vi "数据库1操作.vi"(1 "模糊查找内容":string) -> ()   [LabVIEW 2018]
uses:
  <vilib>/Utility/file.llb/Write To Spreadsheet File (string).vi
panel:
  out "error out 3":errorcluster
  out "error out 2":errorcluster
  in  "选项卡控件":enum32{"读取", "写入", "其他"}(tab)
  in  "保存":bool
  in  "查找":bool
  out "Table":string[][](table) caption="表格"
  in  "查找项目":u16(ring) items=["编号", "名称", "零件号", "图号", "批号"]
  in  "数据库所在位置":path
  in  "userID":string="admin"
  in  "userPWD":string="admin"
  in  "以编号写其他":bool
  in  "时间":string="000007"
  in  "批号":string="000006"
  in  "数量":string="000005"
  in  "图号":string="000004"
  in  "零件号":string="000003"
  in  "名称":string="000002"
  in  "插入编号":string="000001"
  in  "插入编号":bool
  out "error out":errorcluster
  # "vi所在文件夹"
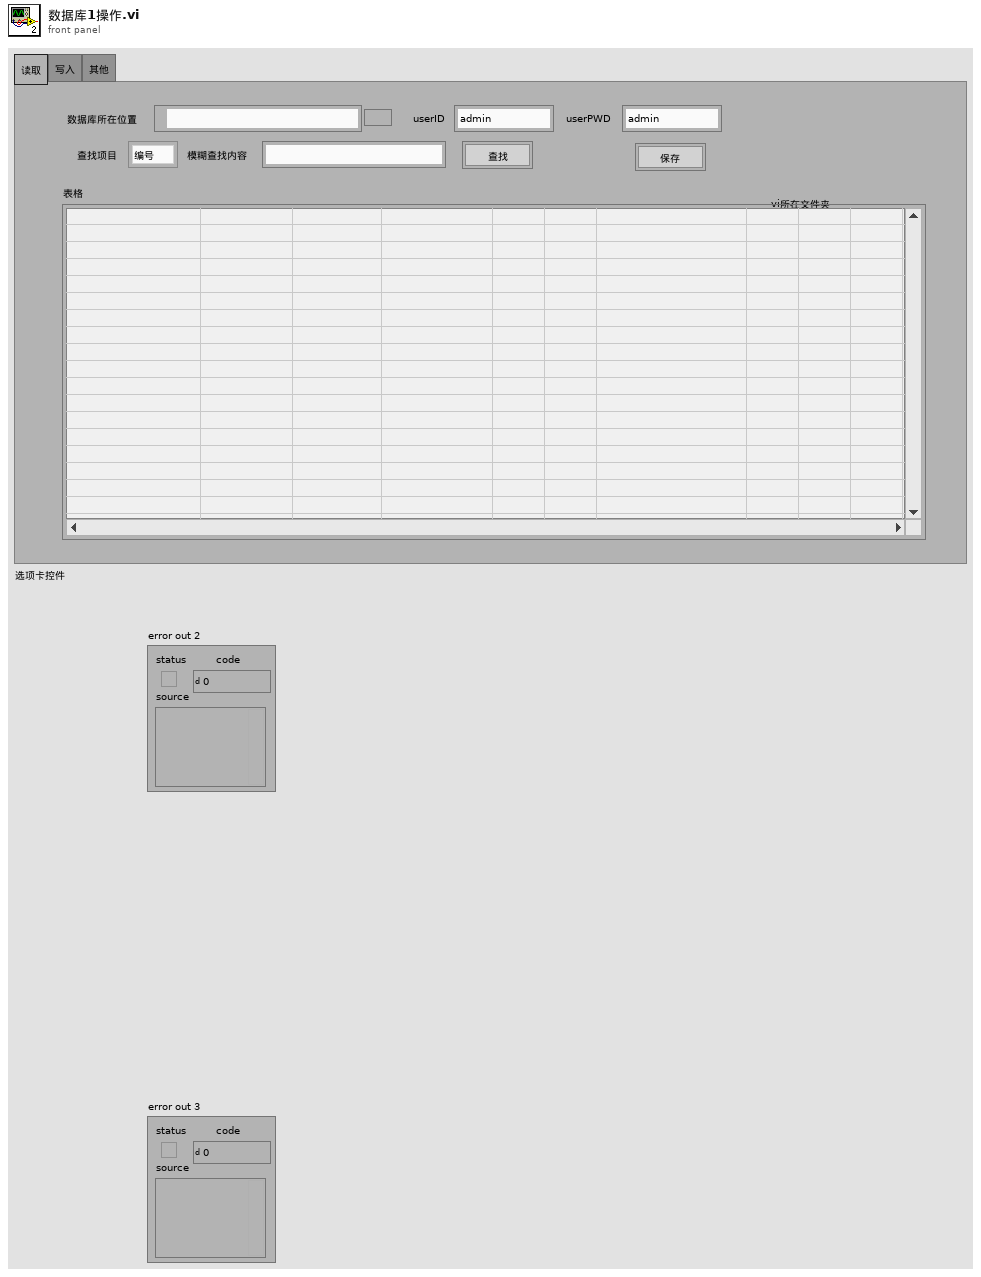
[diagram p1: front panel]
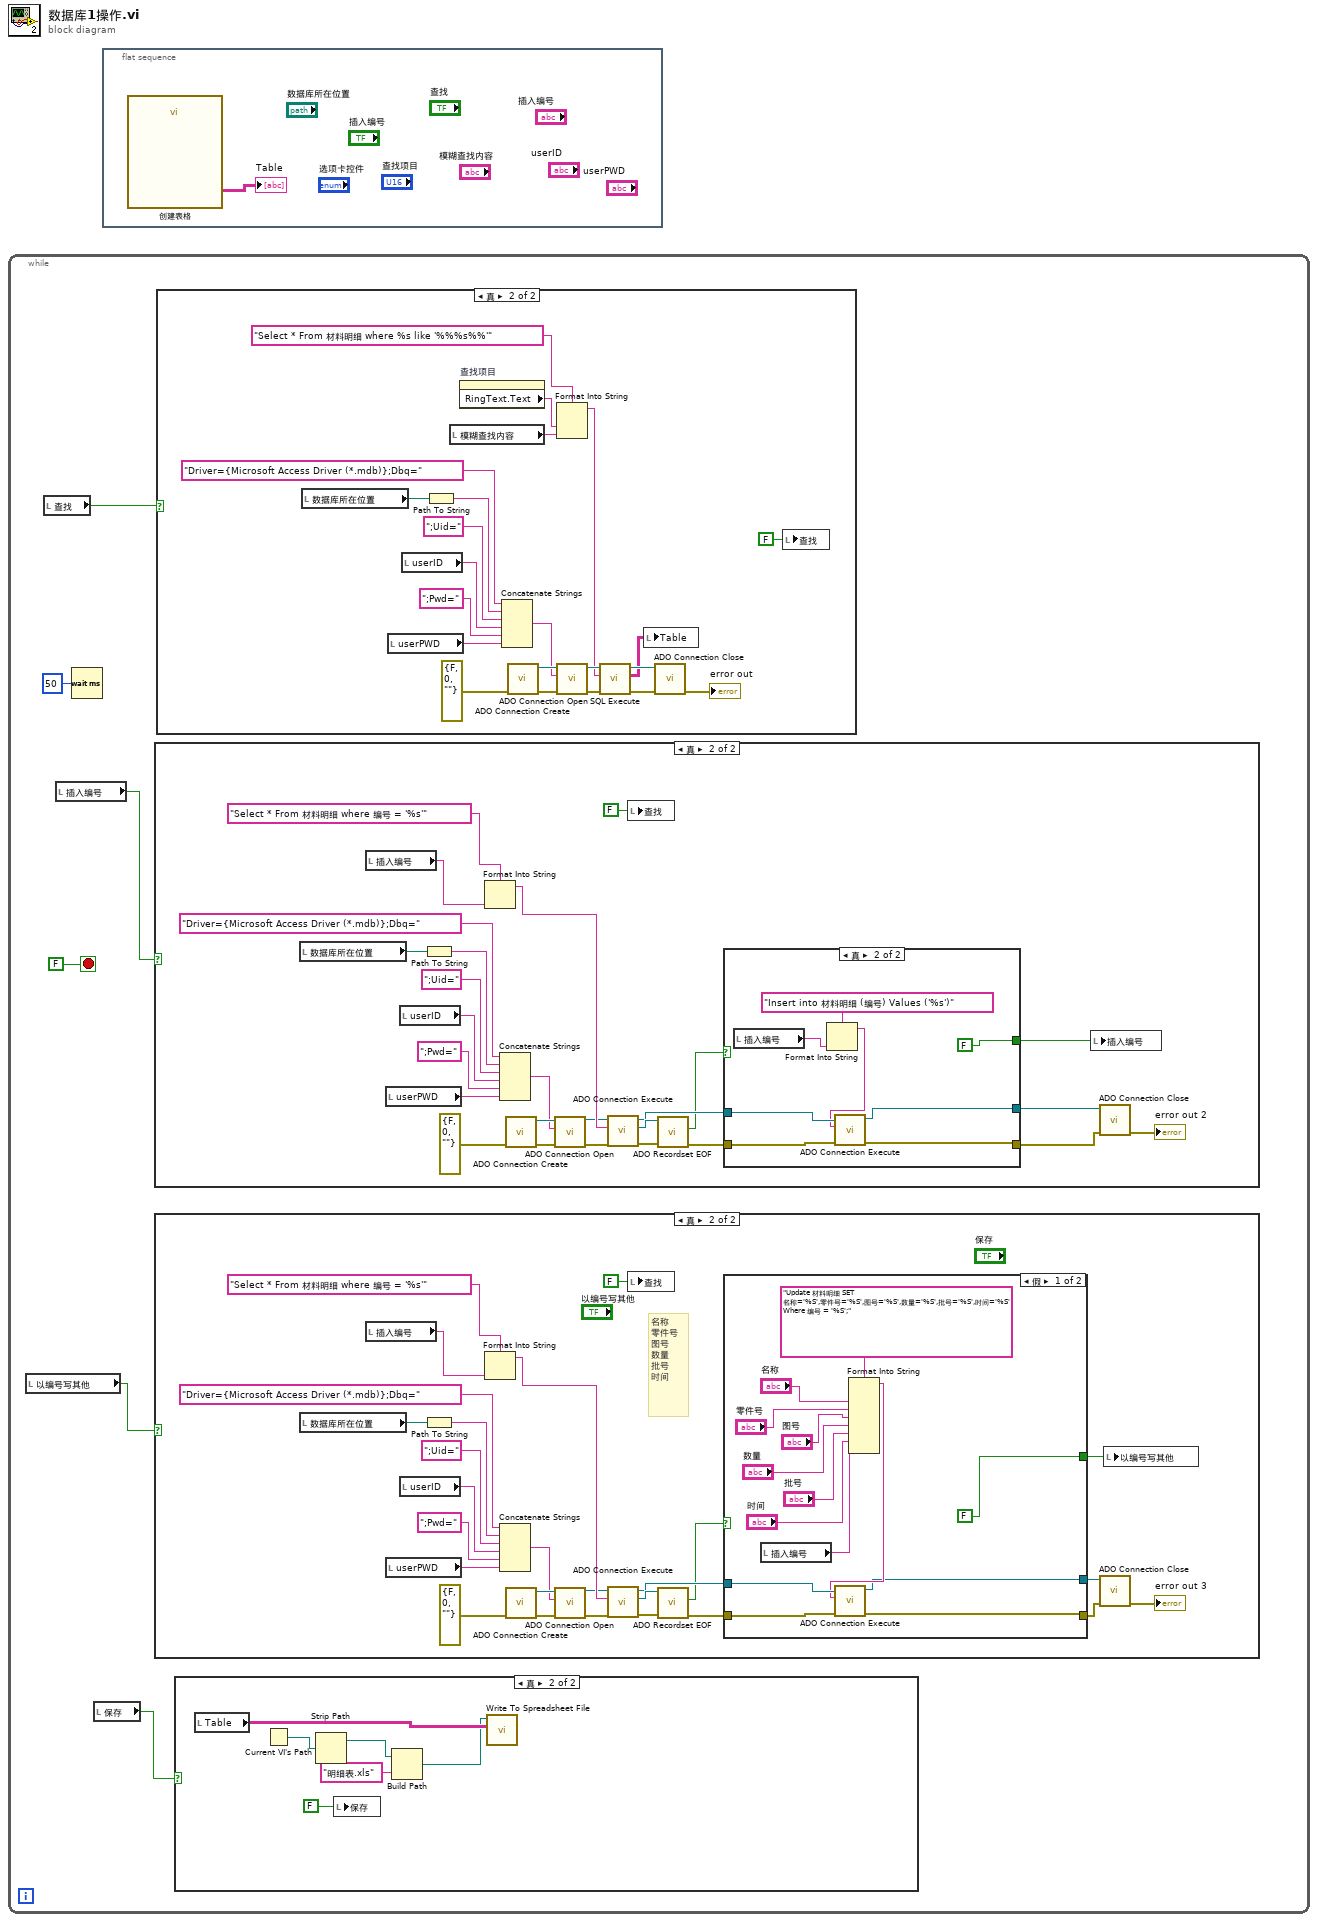
[diagram p0: block diagram]
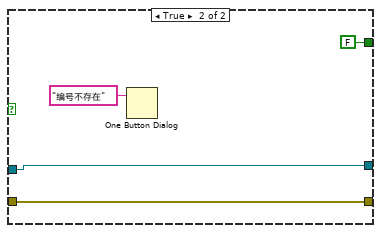
[diagram p4: hidden frame]
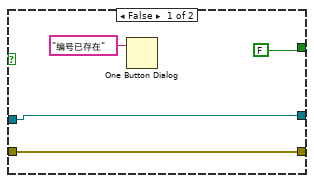
[diagram p6: hidden frame]
diagram:
  n1 = while {
    stop <- FALSE stop-if-true
    n2 = local read "以编号写其他"() -> (w2:bool)
    n3 = local read "查找"() -> (w6:bool)
    n4 = local read "插入编号"() -> (w3:bool)
    n5 = Wait (ms)(milliseconds to wait=u32 50 ("等待时间（毫秒）")) -> ()  [unwired: 1 out]
    n6 = local read "保存"() -> (w1:bool)
    n7 = case shown="真" w3 {
      frame False {
      }
      frame True {
        n8 = local read "数据库所在位置"() -> (w72:path)
        n9 = local read "插入编号"() -> (w68:string)
        n10 = local read "userPWD"() -> (w71:string)
        n11 = local read "userID"() -> (w73:string)
        n12 = Path To String(path=w72) -> (string=w76:string)
        n13 = Format Into String(format string="Select * From 材料明细 where 编号 = '%s'" ("格式字符串"), w68) -> (resulting string=w67:string)  [unwired: 2 in, 1 out]
        n14 = Concatenate Strings("Driver={Microsoft Access Driver (*.mdb)};Dbq=", w76, ";Uid=", w73, ";Pwd=", w71) -> (w77:string)
        n15 = call "ADO Connection Create.vi"("error in (no error)"=errorcluster {"status"=FALSE, "code"=0, "source"=""}) -> ("error out"=w81:errorcluster, "ADODB._Connection Out"=w82:refnum<k7>)  [unwired: 9 out]
        n16 = call "ADO Connection Open.vi"("error in (no error)"=w81, "ConnectionString"=w77, "ADODB._Connection In"=w82) -> ("error out"=w64:errorcluster, "ADODB._Connection Out"=w66:refnum<k7>)  [unwired: 7 out]
        n17 = call "ADO Connection Execute.vi"("error in (no error)"=w64, "CommandText"=w67, "ADODB._Connection In"=w66) -> ("error out"=w63:errorcluster, "RecordSet"=w65:refnum<k7>, "ADODB._Connection Out"=w61:refnum<k7>)  [unwired: 6 in]
        n18 = local write "查找"(FALSE ("读取")) -> ()
        n19 = call "ADO Recordset EOF.vi"("error in (no error)"=w63, "ADODB._Recordset In"=w65) -> ("error out"=w62:errorcluster, "EOF"=w60:bool)  [unwired: 7 in, 1 out]
        n20 = case shown="真" w60 {
          tunnel: w62 -> [w85 w93]
          tunnel: w61 -> [w86 w92]
          tunnel: [w86 w90] -> w59
          tunnel: [w85 w89] -> w58
          tunnel: [FALSE FALSE] -> w57
          frame False {
            n21 = One Button Dialog(message="编号已存在" ("消息")) -> ()  [unwired: 1 in, 1 out]
          }
          frame True {
            n22 = local read "插入编号"() -> (w88:string)
            n23 = Format Into String(format string="Insert into 材料明细 (编号) Values ('%s')" ("格式字符串"), w88) -> (resulting string=w91:string)  [unwired: 2 in, 1 out]
            n24 = call "ADO Connection Execute.vi"("error in (no error)"=w93, "CommandText"=w91, "ADODB._Connection In"=w92) -> ("error out"=w89:errorcluster, "ADODB._Connection Out"=w90:refnum<k7>)  [unwired: 6 in, 1 out]
          }
        }
        n25 = local write "插入编号"(w57) -> ()
        n26 = call "ADO Connection Close.vi"("error in (no error)"=w58, "ADODB._Connection In"=w59) -> ("error out"=→"error out 2":errorcluster)  [unwired: 9 out]
      }
    }
    n27 = case shown="真" w2 {
      frame False {
      }
      frame True {
        # "名称\n零件号\n图号\n数量\n批号\n时间"
        n28 = local read "数据库所在位置"() -> (w28:path)
        n29 = local read "插入编号"() -> (w24:string)
        n30 = local read "userPWD"() -> (w27:string)
        n31 = local read "userID"() -> (w29:string)
        n32 = Path To String(path=w28) -> (string=w32:string)
        n33 = Format Into String(format string="Select * From 材料明细 where 编号 = '%s'" ("格式字符串"), w24) -> (resulting string=w23:string)  [unwired: 2 in, 1 out]
        n34 = Concatenate Strings("Driver={Microsoft Access Driver (*.mdb)};Dbq=", w32, ";Uid=", w29, ";Pwd=", w27) -> (w33:string)
        n35 = call "ADO Connection Create.vi"("error in (no error)"=errorcluster {"status"=FALSE, "code"=0, "source"=""}) -> ("error out"=w37:errorcluster, "ADODB._Connection Out"=w38:refnum<k7>)  [unwired: 9 out]
        n36 = call "ADO Connection Open.vi"("error in (no error)"=w37, "ConnectionString"=w33, "ADODB._Connection In"=w38) -> ("error out"=w20:errorcluster, "ADODB._Connection Out"=w22:refnum<k7>)  [unwired: 7 out]
        n37 = call "ADO Connection Execute.vi"("error in (no error)"=w20, "CommandText"=w23, "ADODB._Connection In"=w22) -> ("error out"=w19:errorcluster, "RecordSet"=w21:refnum<k7>, "ADODB._Connection Out"=w17:refnum<k7>)  [unwired: 6 in]
        n38 = local write "查找"(FALSE ("读取")) -> ()
        n39 = call "ADO Recordset EOF.vi"("error in (no error)"=w19, "ADODB._Recordset In"=w21) -> ("error out"=w18:errorcluster, "EOF"=w16:bool)  [unwired: 7 in, 1 out]
        n40 = case shown="假" w16 {
          tunnel: w18 -> [w51 w55]
          tunnel: w17 -> [w50 w56]
          tunnel: [w48 w56] -> w15
          tunnel: [w47 w55] -> w14
          tunnel: [FALSE FALSE] -> w13
          frame False {
            n41 = local read "插入编号"() -> (w46:string)
            n42 = Format Into String(format string="Update 材料明细 SET 名称='%S',零件号='%S',图号='%S',数量='%S',批号='%S',时间='%S'Where 编号 = '%S';" ("格式字符串"), "名称", "零件号", "图号", "数量", "批号", "时间", w46) -> (resulting string=w49:string)  [unwired: 2 in, 1 out]
            n43 = call "ADO Connection Execute.vi"("error in (no error)"=w51, "CommandText"=w49, "ADODB._Connection In"=w50) -> ("error out"=w47:errorcluster, "ADODB._Connection Out"=w48:refnum<k7>)  [unwired: 6 in, 1 out]
          }
          frame True {
            n44 = One Button Dialog(message="编号不存在" ("消息")) -> ()  [unwired: 1 in, 1 out]
          }
        }
        n45 = call "ADO Connection Close.vi"("error in (no error)"=w14, "ADODB._Connection In"=w15) -> ("error out"=→"error out 3":errorcluster)  [unwired: 9 out]
        n46 = local write "以编号写其他"(w13) -> ()
      }
    }
    n47 = case shown="真" w6 {
      frame False {
      }
      frame True {
        n48 = local read "数据库所在位置"() -> (w97:path)
        n49 = local read "userPWD"() -> (w96:string)
        n50 = local read "userID"() -> (w98:string)
        n51 = Path To String(path=w97) -> (string=w104:string)
        n52 = local read "模糊查找内容"() -> (w99:string)
        n53 = property on="查找项目" class="Ring (严格)"() -> ("RingText.Text"=w102:string)  [unwired: 2 in, 2 out]
        n54 = Concatenate Strings("Driver={Microsoft Access Driver (*.mdb)};Dbq=", w104, ";Uid=", w98, ";Pwd=", w96) -> (w105:string)
        n55 = call "ADO Connection Create.vi"("error in (no error)"=errorcluster {"status"=FALSE, "code"=0, "source"=""}) -> ("error out"=w115:errorcluster, "ADODB._Connection Out"=w116:refnum<k7>)  [unwired: 9 out]
        n56 = Format Into String(format string="Select * From 材料明细 where %s like '%%%s%%'" ("格式字符串"), w102, w99) -> (resulting string=w109:string)  [unwired: 2 in, 1 out]
        n57 = call "ADO Connection Open.vi"("error in (no error)"=w115, "ConnectionString"=w105, "ADODB._Connection In"=w116) -> ("error out"=w114:errorcluster, "ADODB._Connection Out"=w113:refnum<k7>)  [unwired: 7 out]
        n58 = call "SQL Execute.vi"("error in (no error)"=w114, "Command Text"=w109, "ADODB._Connection In"=w113) -> ("error out"=w110:errorcluster, "Data"=w100:string[][], "ADODB._Connection Out"=w112:refnum<k7>)  [unwired: 5 in, 1 out]
        n59 = local write "Table"(w100) -> ()
        n60 = call "ADO Connection Close.vi"("error in (no error)"=w110, "ADODB._Connection In"=w112) -> ("error out"=→"error out":errorcluster)  [unwired: 9 out]
        n61 = local write "查找"(FALSE ("读取")) -> ()
      }
    }
    n62 = case shown="真" w1 {
      frame False {
      }
      frame True {
        n63 = local read "Table"() -> (w12:string[][])
        n64 = Current VI's Path() -> (path=w10:path)
        n65 = Strip Path(path=w10) -> (stripped path=w9:path)  [unwired: 1 out]
        n66 = local write "保存"(FALSE ("另存为")) -> ()
        n67 = Build Path(base path=w9, name or relative path="明细表.xls" ("名称或相对路径")) -> (appended path=w7:path)
        n68 = call-poly <vilib>:"Write To Spreadsheet File.vi"("2D data"=w12, "file path (dialog if empty)"=w7) -> ()  [unwired: 6 in, 1 out]
      }
    }
  }
  n69 = flat-sequence {
    frame #0 {
      n70 = call "创建表格"() -> ("Table"=→"Table":string[][])  [unwired: 5 in, 6 out]
    }
  }
